vi "Export File - Main XML.vi"(6 "RootNode":refnum<k24>, 7 "Import/Export Data - Main":T1, 8 "error in (no error)":errorcluster, 11 "XmlDocument in":refnum<k24>) -> (0 "error out":errorcluster, 3 "XmlDocument out":refnum<k24>)   [LabVIEW 2019, in "UDP-Custom-Device System Explorer.lvlib"]
uses:
  UDP-Custom-Device System Explorer.lvlib
  Types/XML - New/ImpExp - Main Data.ctl
  <vilib>/NI VeriStand/Custom Device API/Custom Device Item Info.ctl
  System.Xml
  <vilib>/NI VeriStand/Custom Device API/Custom Device API.lvlib
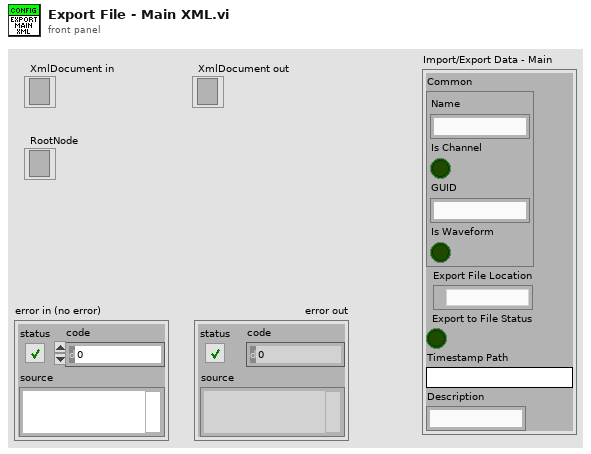
[diagram p1: front panel]
types:
  T1 = typedef "UDP-Custom-Device System Explorer.lvlib/ImpExp - Main Data.ctl" = cluster{"Common":T2, "Export File Location":path, "Export to File Status":bool, "Timestamp Path":string, "Description":string}
  T2 = typedef "Custom Device API.lvlib/Custom Device Item Info.ctl" = cluster{"Name":string, "Is Channel":bool, "GUID":string, "Is Waveform":bool}
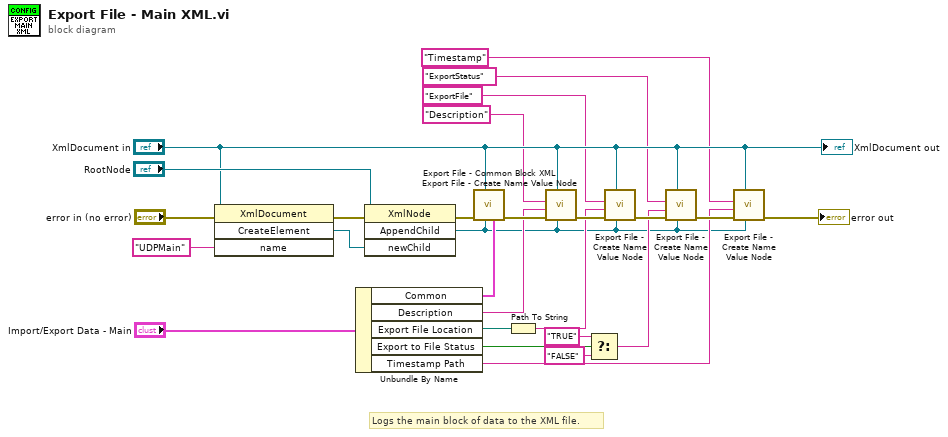
[diagram p0: block diagram]
diagram:
  # "Logs the main block of data to the XML file."
  n1 = invoke class="XmlDocument" method="CreateElement"(reference="XmlDocument in", error in="error in (no error)", "name"="UDPMain" ("Tag Name")) -> (error out=w22:errorcluster, "CreateElement"=w23:refnum<k24>)  [unwired: 1 in, 2 out]
  n2 = Unbundle By Name("Import/Export Data - Main") -> ("Common"=w14:T2, "Description"=w13:string, "Export File Location"=w8:path, "Export to File Status"=w10:bool, "Timestamp Path"=w3:string)
  n3 = invoke class="XmlNode" method="AppendChild"(reference="RootNode", error in=w22, "newChild"=w23) -> (error out=w21:errorcluster, "AppendChild"=w1:refnum<k24>)  [unwired: 1 in, 2 out]
  n4 = call "Export File - Common Block XML.vi"("Common"=w14, "RootNode in"=w1, "XmlDocument in"="XmlDocument in", "error in (no error)"=w21) -> ("error out"=w17:errorcluster)  [unwired: 7 in]
  n5 = Path To String(path=w8) -> (string=w7:string)
  n6 = call "Export File - Create Name Value Node.vi"("RootNode in"=w1, "XmlDocument in"="XmlDocument in", "error in (no error)"=w17, "Value"=w13, "Name"="Description" ("name")) -> ("error out"=w20:errorcluster)  [unwired: 6 in]
  n7 = Select(t="TRUE" ("name"), s=w10, f="FALSE" ("name")) -> (s? t:f=w9:string)
  n8 = call "Export File - Create Name Value Node.vi"("RootNode in"=w1, "XmlDocument in"="XmlDocument in", "error in (no error)"=w20, "Value"=w7, "Name"="ExportFile" ("name")) -> ("error out"=w19:errorcluster)  [unwired: 6 in]
  n9 = call "Export File - Create Name Value Node.vi"("RootNode in"=w1, "XmlDocument in"="XmlDocument in", "error in (no error)"=w19, "Value"=w9, "Name"="ExportStatus" ("name")) -> ("error out"=w18:errorcluster)  [unwired: 6 in]
  n10 = call "Export File - Create Name Value Node.vi"("RootNode in"=w1, "XmlDocument in"="XmlDocument in", "error in (no error)"=w18, "Value"=w3, "Name"="Timestamp" ("name")) -> ("error out"=→"error out":errorcluster)  [unwired: 6 in]
  "XmlDocument out" <- "XmlDocument in"
